vi "TiMicSDK.vi"() -> ()   [LabVIEW 2011]
uses:
  TILLPhotonics/DevID.ctl
panel:
  out "Value":string
  out "error out":errorcluster
  out "command":string
  # "version without z"
  # "*.z=\"1..\"\n*.x=\"...\"\n*.y=\"...\"\n*.f1=\"..\"\n*.turret=\"...\"\njeweils .set werte"
  # "stage.x.set=\"update\" for read"
  # "remember state! arrival time? not to sent new command before arrival!"
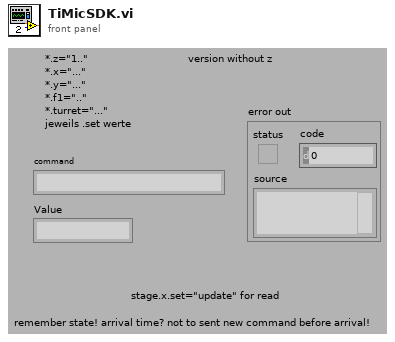
[diagram p1: front panel]
types:
  T1 = enum16{"None/#Datasets", "Clear", "TagValueOf#", "AddValues", "ReadValue", "ChangeValue", "Get all"}
  T2 = typedef "DevID.ctl" = i32
  T3 = enum16{"no error", "missing axis", "missing Z axis", "missing Filter", "iMic not initialized", "no property", "wrong handle", "protocol not finished", "user parameter to long (>32 bits)", "no user parameter handle", "failed to open comport", "failed to initialize"}
  T4 = cluster{bool, "output param":enum16{"no error", "missing axis", "missing Z axis", "missing Filter", "iMic not initialized", "no property", "wrong handle", "protocol not finished", "user parameter to long (>32 bits)", "no user parameter handle", "failed to open comport", "failed to initialize"}, string}
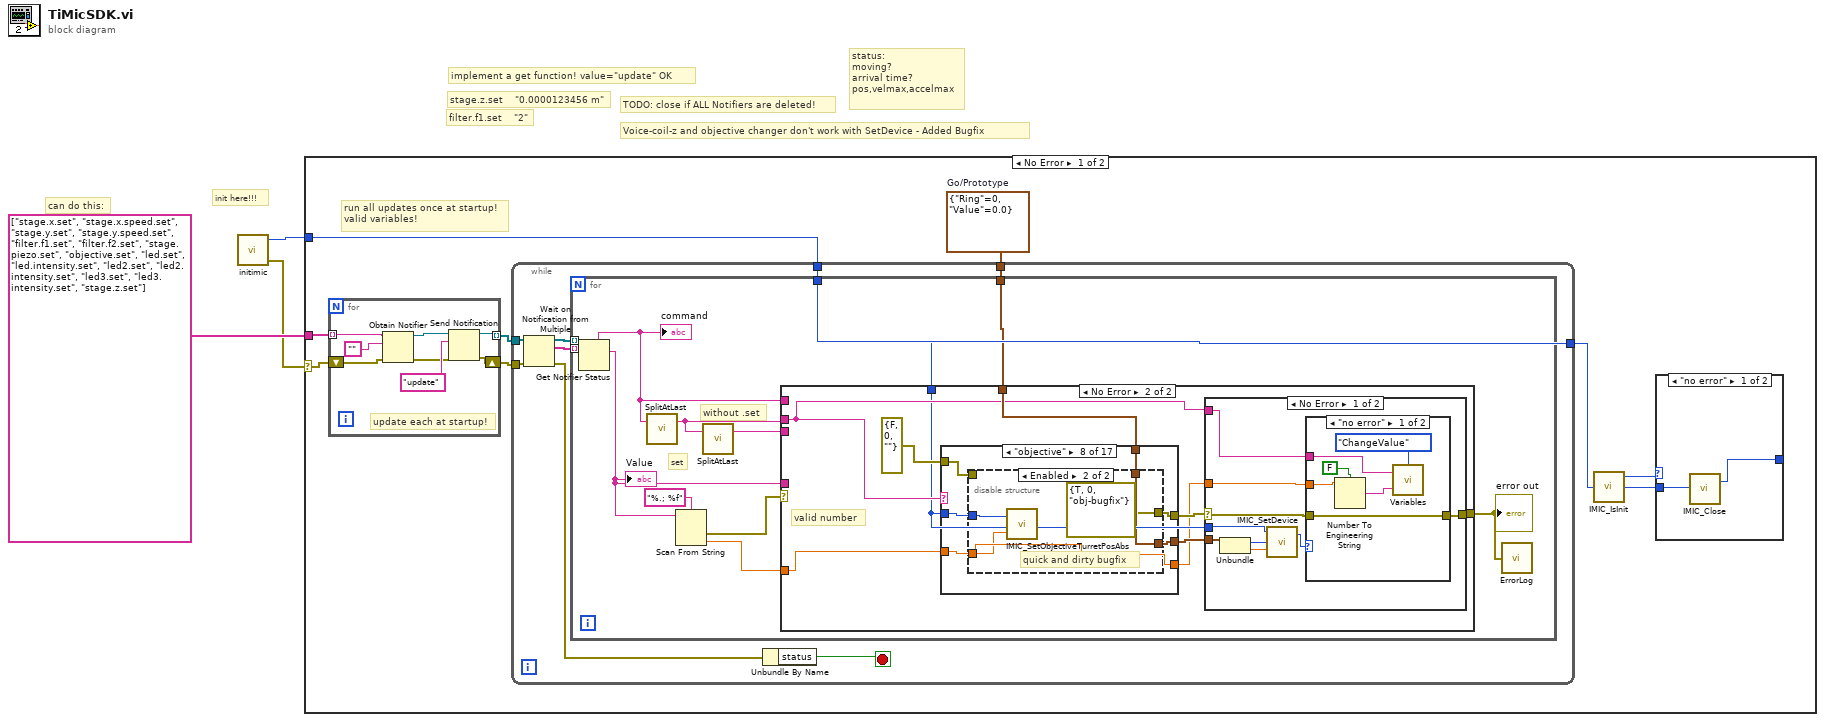
[diagram p0: block diagram]
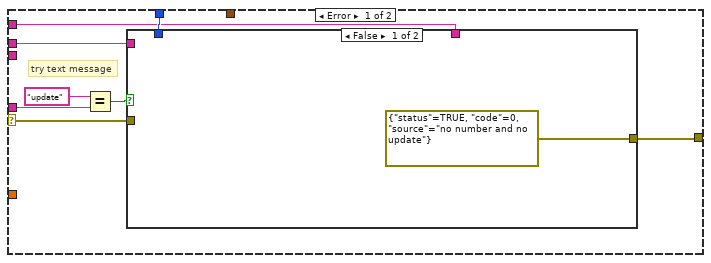
[diagram p3: hidden frame]
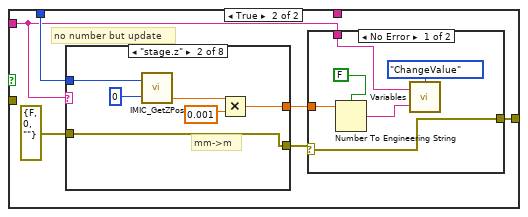
[diagram p4: hidden frame]
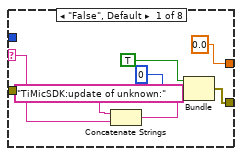
[diagram p6: hidden frame]
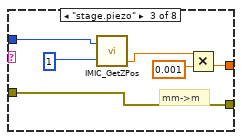
[diagram p7: hidden frame]
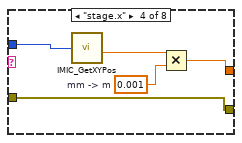
[diagram p8: hidden frame]
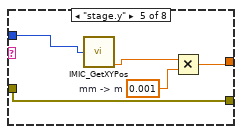
[diagram p9: hidden frame]
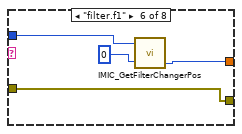
[diagram p10: hidden frame]
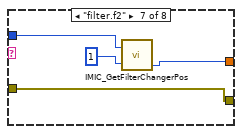
[diagram p11: hidden frame]
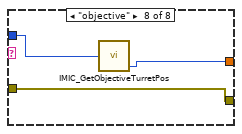
[diagram p12: hidden frame]
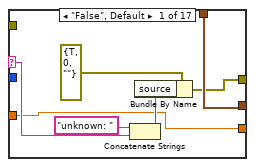
[diagram p13: hidden frame]
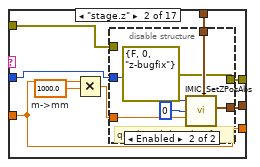
[diagram p14: hidden frame]
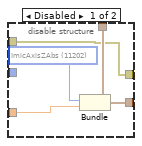
[diagram p15: hidden frame]
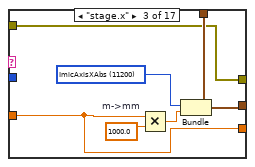
[diagram p16: hidden frame]
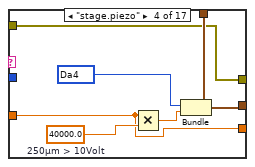
[diagram p17: hidden frame]
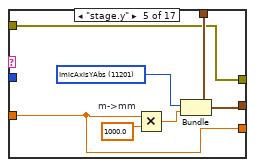
[diagram p18: hidden frame]
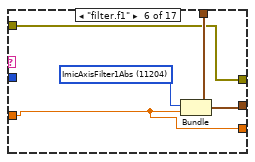
[diagram p19: hidden frame]
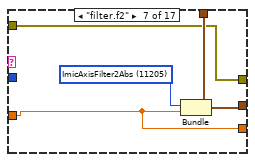
[diagram p20: hidden frame]
diagram:
  # "can do this:"
  # "Voice-coil-z and objective changer don't work with SetDevice - Added Bugfix"
  # "filter.f1.set    \"2\""
  # "status:\nmoving?\narrival time?\npos,velmax,accelmax"
  # "implement a get function! value=\"update\" OK"
  # "TODO: close if ALL Notifiers are deleted!"
  # "init here!!!"
  # "stage.z.set    \"0.0000123456 m\""
  n1 = call "initimic.vi"() -> ("handle"=w3:u64, "error out"=w1:errorcluster)  [unwired: 3 out]
  n2 = case shown="No Error" w1 {
    selector: w1 -> [w4 _]
    tunnel: w3 -> [w12 _]
    tunnel: string[] ["stage.x.set", "stage.x.speed.set", "stage.y.set", "stage.y.speed.set", "filter.f1.set", "filter.f2.set", "stage.piezo.set", "objective.set", "led.set", "led.intensity.set", "led2.set", "led2.intensity.set", "led3.set", "led3.intensity.set", "stage.z.set"] -> [w7 _]
    frame No Error {
      w8 = cluster{"Ring":T2, "Value":dbl} {"Ring"=0, "Value"=0.0}  # Go/Prototype
      # "run all updates once at startup!\nvalid variables!"
      n3 = for {
        tunnel: w7 -> [w20] mode=indexing
        tunnel: [w14] -> w6 mode=indexing
        shift-right: [w13] -> w5
        shift-left: w4 -> [w18]
        # "update each at startup!"
        n4 = Obtain Notifier(name (unnamed)=w20, notification data type="", error in (no error)=w18) -> (notifier out=w16:refnum<notifier>, error out=w15:errorcluster)  [unwired: 1 in, 1 out]
        n5 = Send Notification(notification="update" ("Meldung"), notifier=w16, error in (no error)=w15) -> (notifier out=w14:refnum<notifier>, error out=w13:errorcluster)
      }
      n6 = while {
        tunnel: w6 -> [w26]
        tunnel: w12 -> [w30]
        tunnel: w5 -> [w28]
        tunnel: [w30] -> w10
        tunnel: w8 -> [w29]
        stop <- w31 stop-if-true
        n7 = Wait on Notification from Multiple(0:w26, 3:w28) -> (8:w25:refnum<notifier>[], 9:w24:string[], 11:w27:errorcluster)  [unwired: 3 out]
        n8 = for {
          tunnel: w30 -> [w42]
          tunnel: w29 -> [w41]
          tunnel: w25 -> [w40] mode=indexing
          tunnel: w24 -> [_] mode=indexing
          # "without .set"
          # "set"
          n9 = Get Notifier Status(notifier=w40) -> (notifier name=w39:string, current notification=w33:string)  [unwired: 1 in, 3 out]
          "command" <- w39
          "Value" <- w33
          n10 = call "SplitAtLast.vi"("In-String"=w39) -> ("Front (default)"=w38:string)  [unwired: 1 in, 1 out]
          n11 = Scan From String(format string="%.; %f", input string=w33) -> (error out=w34:errorcluster, output 1=w35:dbl)  [unwired: 2 in, 3 out]
          n12 = call "SplitAtLast.vi"("In-String"=w38) -> ("Front (default)"=w37:string)  [unwired: 1 in, 1 out]
          n13 = case shown="No Error" w34 {
            selector: w34 -> [w48 _]
            tunnel: [w49 w113] -> w32
            tunnel: w42 -> [w50 w107]
            tunnel: w38 -> [w43 w108]
            tunnel: w39 -> [w47 _]
            tunnel: w41 -> [_ w111]
            tunnel: w37 -> [_ _]
            tunnel: w35 -> [_ w106]
            tunnel: w33 -> [w46 _]
            frame Error {
              # "try text message"
              n14 = Equal?(x="update", y=w46) -> (x = y?=w44:bool)
              n15 = case shown="False" w44 {
                tunnel: w50 -> [_ w57]
                tunnel: [errorcluster {"status"=TRUE, "code"=0, "source"="no number and no update"} ("error out") w56] -> w49
                tunnel: w48 -> [_ _]
                tunnel: w47 -> [_ _]
                tunnel: w43 -> [_ w54]
                frame False {
                }
                frame True {
                  # "no number but update"
                  n16 = case shown="\"stage.z\"" w54 {
                    selector: w54 -> [w69 _ _ _ _ _ _ _]
                    tunnel: w57 -> [_ w77 w83 w88 w92 w97 w100 w104]
                    tunnel: [0.0 ("zpos") w73 w79 w85 w90 w95 w99 w103] -> w55
                    tunnel: errorcluster {"status"=FALSE, "code"=0, "source"=""} ("error out") -> [_ w72 w78 w84 w89 w94 w98 w102]
                    tunnel: [w68 w72 w78 w84 w89 w94 w98 w102] -> w52
                    frame "False", Default {
                      n17 = Concatenate Strings("TiMicSDK:update of unknown:" ("source"), w69) -> (w65:string)
                      n18 = Bundle("status"=TRUE, "code"=0, w65) -> (w68:cluster{"status":bool, "code":i32, string})  [unwired: 1 out]
                    }
                    frame "stage.z" {
                      # "mm->m"
                      n19 = call "IMIC_GetZPos.vi"("handle"=w77, "index"=0) -> ("zpos"=w74:dbl)  [unwired: 2 out]
                      n20 = Multiply(x=w74, y=0.001) -> (x*y=w73:dbl)
                    }
                    frame "stage.piezo" {
                      # "mm->m"
                      n21 = call "IMIC_GetZPos.vi"("handle"=w83, "index"=1) -> ("zpos"=w80:dbl)  [unwired: 2 out]
                      n22 = Multiply(x=w80, y=0.001) -> (x*y=w79:dbl)
                    }
                    frame "stage.x" {
                      w86 = 0.001  # mm -> m
                      n23 = call "IMIC_GetXYPos.vi"("handle"=w88) -> ("xpos"=w87:dbl)  [unwired: 3 out]
                      n24 = Multiply(x=w87, y=w86) -> (x*y=w85:dbl)
                    }
                    frame "stage.y" {
                      w93 = 0.001  # mm -> m
                      n25 = call "IMIC_GetXYPos.vi"("handle"=w92) -> ("ypos"=w91:dbl)  [unwired: 3 out]
                      n26 = Multiply(x=w91, y=w93) -> (x*y=w90:dbl)
                    }
                    frame "filter.f1" {
                      n27 = call "IMIC_GetFilterChangerPos.vi"("handle"=w97, "index"=0) -> ("Filter"=w95:i32)  [unwired: 2 out]
                    }
                    frame "filter.f2" {
                      n28 = call "IMIC_GetFilterChangerPos.vi"("handle"=w100, "index"=1) -> ("Filter"=w99:i32)  [unwired: 2 out]
                    }
                    frame "objective" {
                      n29 = call "IMIC_GetObjectiveTurretPos.vi"("handle"=w104) -> ("Objective"=w103:i32)  [unwired: 2 out]
                    }
                  }
                  n30 = case shown="No Error" w52 {
                    selector: w52 -> [w58 w64]
                    tunnel: [w58 w64] -> w56
                    tunnel: w55 -> [w60 _]
                    tunnel: w54 -> [w59 _]
                    frame No Error {
                      n31 = Number To Engineering String(1:FALSE ("use system decimal point (T)"), 4:w60) -> (0:w63:string)  [unwired: 2 out]
                      n32 = call "Variables.vi"("value"=w63, "Tag in"=w59, "Command"=T1."ChangeValue") -> ()  [unwired: 3 out]
                    }
                    frame Error {
                    }
                  }
                }
              }
            }
            frame No Error {
              # "valid number"
              n33 = case shown="\"objective\"" w108 {
                selector: w108 -> [w118 _ _ _ _ _ _ _ _ _ _ _ _ _ _ _ _]
                tunnel: w106 -> [w114 w125 w139 w146 w153 w160 w165 w172 w185 w195 w205 w219 w228 w236 w243 w251 w260]
                tunnel: [w115 w122 w141 w149 w155 w161 w166 w170 w187 w196 w206 w215 w224 w232 w239 w247 w256] -> w109
                tunnel: [w120 w126 w143 w151 w157 w163 w168 w175 w188 w198 w207 w222 w230 w238 w241 w249 w258] -> w110
                tunnel: w111 -> [w120 w127 w144 w152 w158 w164 w169 w173 w186 w197 w208 w221 w229 w237 w240 w248 w257]
                tunnel: errorcluster {"status"=FALSE, "code"=0, "source"=""} ("error in (no error)") -> [_ w123 w141 w149 w155 w161 w166 w171 w187 w196 w206 w215 w224 w232 w239 w247 w256]
                tunnel: w107 -> [_ w121 _ _ _ _ _ w174 _ _ _ _ _ _ _ _ _]
                tunnel: [w114 w125 w139 w146 w153 w160 w165 w172 w185 w195 w205 w216 w225 w233 w242 w250 w259] -> w105
                frame "False", Default {
                  n34 = Concatenate Strings("unknown: ", w118) -> (w117:string)
                  n35 = Bundle By Name(cluster=errorcluster {"status"=TRUE, "code"=0, "source"=""} ("error out"), "source"=w117) -> (w115:errorcluster)
                }
                frame "stage.z" {
                  w128 = 1000.0  # m->mm
                  n36 = Multiply(x=w125, y=w128) -> (x*y=w124:dbl)
                  n37 = disable-structure shown="Enabled" {
                    disable-tunnel: w127 -> [w133 w138]
                    disable-tunnel: [w132 w138] -> w126
                    disable-tunnel: w124 -> [w130 w135]
                    disable-tunnel: w123 -> [w129 _]
                    disable-tunnel: [w129 errorcluster {"status"=FALSE, "code"=0, "source"="z-bugfix"} ("error in (no error)")] -> w122
                    disable-tunnel: w121 -> [_ w136]
                    frame Disabled {
                      w131 = 11202 items=["EndLoop"=-2, "Loop"=-1, "Invalid"=0, "TriggerPolyV"=1, "TriggerCamera"=2, "SyncCamera"=3, "Do1"=1000, "Do2"=1001, "Do3"=1002, "Do4"=1003, "Do5"=1004, "Do6"=1005, "Do7"=1006, "Do8"=1007, "Do9"=1008, "Do10"=1009, "Do11"=1010, "Do12"=1011, "Do13"=1012, "Do14"=1013, "Do15"=1014, "Do16"=1015, "Do17"=1016, "Do18"=1017, "Do19"=1018, "Do20"=1019, "Do21"=1020, "Do22"=1021, "Do23"=1022, "Do24"=1023, "Do_End"=1024, "Da1"=2000, "Da2"=2001, "Da3"=2002, "Da4"=2003, "Da5"=2004, "Da6"=2005, "Da7"=2006, "Da8"=2007, "DaIncr_First"=2008, "Da1Incr"=2100, "Da2Incr"=2101, "Da3Incr"=2102, "Da4Incr"=2103, "Da5Incr"=2104, "Da6Incr"=2105, "Da7Incr"=2106, "Da8Incr"=2107, "Da1Raw"=2200, "Da2Raw"=2201, "Da3Raw"=2202, "Da4Raw"=2203, "Da5Raw"=2204, "Da6Raw"=2205, "Da7Raw"=2206, "Da8Raw"=2207, "Da1RawIncr"=2300, "Da2RawIncr"=2301, "Da3RawIncr"=2302, "Da4RawIncr"=2303, "Da5RawIncr"=2304, "Da6RawIncr"=2305, "Da7RawIncr"=2306, "Da8RawIncr"=2307, "Uart1"=3000, "Uart2"=3001, "Uart3"=3002, "Uart_End"=3003, "Di1"=4000, "Di2"=4001, "Di3"=4002, "Di4"=4003, "Di5"=4004, "Di6"=4005, "Di7"=4006, "Di8"=4007, "Di9"=4008, "Di10"=4009, "Di11"=4010, "Di12"=4011, "Di13"=4012, "Di14"=4013, "Di15"=4014, "Di16"=4015, "Di17"=4016, "Di18"=4017, "Di19"=4018, "Di20"=4019, "Di21"=4020, "Di22"=4021, "Di23"=4022, "Di24"=4023, "Di_End"=4024, "ICU_End"=4025, "LedIllum"=10000, "ImicAxisXRel"=11000, "ImicAxisYRel"=11001, "ImicAxisZRel"=11002, "ImicAxisTurretRel"=11003, "ImicAxisFilter1Rel"=11004, "ImicAxisFilter2Rel"=11005, "ImicAxis_End"=11006, "ImicAxisXAbs"=11200, "ImicAxisYAbs"=11201, "ImicAxisZAbs"=11202, "ImicAxisTurretAbs"=11203, "ImicAxisFilter1Abs"=11204, "ImicAxisFilter2Abs"=11205, "ImicAxisXVel"=11300, "ImicAxisYVel"=11301, "ImicAxisZVel"=11302, "ImicAxisTurretVel"=11303, "ImicAxisFilter1Vel"=11304, "ImicAxisFilter2Vel"=11305, "ImicAxisXMoving"=11400, "ImicAxisYMoving"=11401, "ImicAxisZMoving"=11402, "ImicAxisTurretMoving"=11403, "ImicAxisFilter1Moving"=11404, "ImicAxisFilter2Moving"=11405, "ImicPiezoClip"=12001, "ImicPiezo"=12002, "IMIC_End"=12003] ("DeviceID")
                      n38 = Bundle(cluster=w133, "Ring"=w131, "Value"=w130) -> (w132:cluster{"Ring":T2, "Value":dbl})
                    }
                    frame Enabled {
                      # "quick and dirty bugfix"
                      n39 = call "IMIC_SetZPosAbs.vi"("zpos"=w135, "index"=0, "handle"=w136) -> ()  [unwired: 2 out]
                    }
                  }
                }
                frame "stage.x" {
                  w142 = 11200 items=["EndLoop"=-2, "Loop"=-1, "Invalid"=0, "TriggerPolyV"=1, "TriggerCamera"=2, "SyncCamera"=3, "Do1"=1000, "Do2"=1001, "Do3"=1002, "Do4"=1003, "Do5"=1004, "Do6"=1005, "Do7"=1006, "Do8"=1007, "Do9"=1008, "Do10"=1009, "Do11"=1010, "Do12"=1011, "Do13"=1012, "Do14"=1013, "Do15"=1014, "Do16"=1015, "Do17"=1016, "Do18"=1017, "Do19"=1018, "Do20"=1019, "Do21"=1020, "Do22"=1021, "Do23"=1022, "Do24"=1023, "Do_End"=1024, "Da1"=2000, "Da2"=2001, "Da3"=2002, "Da4"=2003, "Da5"=2004, "Da6"=2005, "Da7"=2006, "Da8"=2007, "DaIncr_First"=2008, "Da1Incr"=2100, "Da2Incr"=2101, "Da3Incr"=2102, "Da4Incr"=2103, "Da5Incr"=2104, "Da6Incr"=2105, "Da7Incr"=2106, "Da8Incr"=2107, "Da1Raw"=2200, "Da2Raw"=2201, "Da3Raw"=2202, "Da4Raw"=2203, "Da5Raw"=2204, "Da6Raw"=2205, "Da7Raw"=2206, "Da8Raw"=2207, "Da1RawIncr"=2300, "Da2RawIncr"=2301, "Da3RawIncr"=2302, "Da4RawIncr"=2303, "Da5RawIncr"=2304, "Da6RawIncr"=2305, "Da7RawIncr"=2306, "Da8RawIncr"=2307, "Uart1"=3000, "Uart2"=3001, "Uart3"=3002, "Uart_End"=3003, "Di1"=4000, "Di2"=4001, "Di3"=4002, "Di4"=4003, "Di5"=4004, "Di6"=4005, "Di7"=4006, "Di8"=4007, "Di9"=4008, "Di10"=4009, "Di11"=4010, "Di12"=4011, "Di13"=4012, "Di14"=4013, "Di15"=4014, "Di16"=4015, "Di17"=4016, "Di18"=4017, "Di19"=4018, "Di20"=4019, "Di21"=4020, "Di22"=4021, "Di23"=4022, "Di24"=4023, "Di_End"=4024, "ICU_End"=4025, "LedIllum"=10000, "ImicAxisXRel"=11000, "ImicAxisYRel"=11001, "ImicAxisZRel"=11002, "ImicAxisTurretRel"=11003, "ImicAxisFilter1Rel"=11004, "ImicAxisFilter2Rel"=11005, "ImicAxis_End"=11006, "ImicAxisXAbs"=11200, "ImicAxisYAbs"=11201, "ImicAxisZAbs"=11202, "ImicAxisTurretAbs"=11203, "ImicAxisFilter1Abs"=11204, "ImicAxisFilter2Abs"=11205, "ImicAxisXVel"=11300, "ImicAxisYVel"=11301, "ImicAxisZVel"=11302, "ImicAxisTurretVel"=11303, "ImicAxisFilter1Vel"=11304, "ImicAxisFilter2Vel"=11305, "ImicAxisXMoving"=11400, "ImicAxisYMoving"=11401, "ImicAxisZMoving"=11402, "ImicAxisTurretMoving"=11403, "ImicAxisFilter1Moving"=11404, "ImicAxisFilter2Moving"=11405, "ImicPiezoClip"=12001, "ImicPiezo"=12002, "IMIC_End"=12003] ("DeviceID")
                  w145 = 1000.0  # m->mm
                  n40 = Multiply(x=w139, y=w145) -> (x*y=w140:dbl)
                  n41 = Bundle(cluster=w144, "Ring"=w142, "Value"=w140) -> (w143:cluster{"Ring":T2, "Value":dbl})
                }
                frame "stage.piezo" {
                  w147 = 40000.0  # 250µm > 10Volt
                  w150 = 2003 items=["EndLoop"=-2, "Loop"=-1, "Invalid"=0, "TriggerPolyV"=1, "TriggerCamera"=2, "SyncCamera"=3, "Do1"=1000, "Do2"=1001, "Do3"=1002, "Do4"=1003, "Do5"=1004, "Do6"=1005, "Do7"=1006, "Do8"=1007, "Do9"=1008, "Do10"=1009, "Do11"=1010, "Do12"=1011, "Do13"=1012, "Do14"=1013, "Do15"=1014, "Do16"=1015, "Do17"=1016, "Do18"=1017, "Do19"=1018, "Do20"=1019, "Do21"=1020, "Do22"=1021, "Do23"=1022, "Do24"=1023, "Do_End"=1024, "Da1"=2000, "Da2"=2001, "Da3"=2002, "Da4"=2003, "Da5"=2004, "Da6"=2005, "Da7"=2006, "Da8"=2007, "DaIncr_First"=2008, "Da1Incr"=2100, "Da2Incr"=2101, "Da3Incr"=2102, "Da4Incr"=2103, "Da5Incr"=2104, "Da6Incr"=2105, "Da7Incr"=2106, "Da8Incr"=2107, "Da1Raw"=2200, "Da2Raw"=2201, "Da3Raw"=2202, "Da4Raw"=2203, "Da5Raw"=2204, "Da6Raw"=2205, "Da7Raw"=2206, "Da8Raw"=2207, "Da1RawIncr"=2300, "Da2RawIncr"=2301, "Da3RawIncr"=2302, "Da4RawIncr"=2303, "Da5RawIncr"=2304, "Da6RawIncr"=2305, "Da7RawIncr"=2306, "Da8RawIncr"=2307, "Uart1"=3000, "Uart2"=3001, "Uart3"=3002, "Uart_End"=3003, "Di1"=4000, "Di2"=4001, "Di3"=4002, "Di4"=4003, "Di5"=4004, "Di6"=4005, "Di7"=4006, "Di8"=4007, "Di9"=4008, "Di10"=4009, "Di11"=4010, "Di12"=4011, "Di13"=4012, "Di14"=4013, "Di15"=4014, "Di16"=4015, "Di17"=4016, "Di18"=4017, "Di19"=4018, "Di20"=4019, "Di21"=4020, "Di22"=4021, "Di23"=4022, "Di24"=4023, "Di_End"=4024, "ICU_End"=4025, "LedIllum"=10000, "ImicAxisXRel"=11000, "ImicAxisYRel"=11001, "ImicAxisZRel"=11002, "ImicAxisTurretRel"=11003, "ImicAxisFilter1Rel"=11004, "ImicAxisFilter2Rel"=11005, "ImicAxis_End"=11006, "ImicAxisXAbs"=11200, "ImicAxisYAbs"=11201, "ImicAxisZAbs"=11202, "ImicAxisTurretAbs"=11203, "ImicAxisFilter1Abs"=11204, "ImicAxisFilter2Abs"=11205, "ImicAxisXVel"=11300, "ImicAxisYVel"=11301, "ImicAxisZVel"=11302, "ImicAxisTurretVel"=11303, "ImicAxisFilter1Vel"=11304, "ImicAxisFilter2Vel"=11305, "ImicAxisXMoving"=11400, "ImicAxisYMoving"=11401, "ImicAxisZMoving"=11402, "ImicAxisTurretMoving"=11403, "ImicAxisFilter1Moving"=11404, "ImicAxisFilter2Moving"=11405, "ImicPiezoClip"=12001, "ImicPiezo"=12002, "IMIC_End"=12003] ("DeviceID")
                  n42 = Multiply(x=w146, y=w147) -> (x*y=w148:dbl)
                  n43 = Bundle(cluster=w152, "Ring"=w150, "Value"=w148) -> (w151:cluster{"Ring":T2, "Value":dbl})
                }
                frame "stage.y" {
                  w156 = 11201 items=["EndLoop"=-2, "Loop"=-1, "Invalid"=0, "TriggerPolyV"=1, "TriggerCamera"=2, "SyncCamera"=3, "Do1"=1000, "Do2"=1001, "Do3"=1002, "Do4"=1003, "Do5"=1004, "Do6"=1005, "Do7"=1006, "Do8"=1007, "Do9"=1008, "Do10"=1009, "Do11"=1010, "Do12"=1011, "Do13"=1012, "Do14"=1013, "Do15"=1014, "Do16"=1015, "Do17"=1016, "Do18"=1017, "Do19"=1018, "Do20"=1019, "Do21"=1020, "Do22"=1021, "Do23"=1022, "Do24"=1023, "Do_End"=1024, "Da1"=2000, "Da2"=2001, "Da3"=2002, "Da4"=2003, "Da5"=2004, "Da6"=2005, "Da7"=2006, "Da8"=2007, "DaIncr_First"=2008, "Da1Incr"=2100, "Da2Incr"=2101, "Da3Incr"=2102, "Da4Incr"=2103, "Da5Incr"=2104, "Da6Incr"=2105, "Da7Incr"=2106, "Da8Incr"=2107, "Da1Raw"=2200, "Da2Raw"=2201, "Da3Raw"=2202, "Da4Raw"=2203, "Da5Raw"=2204, "Da6Raw"=2205, "Da7Raw"=2206, "Da8Raw"=2207, "Da1RawIncr"=2300, "Da2RawIncr"=2301, "Da3RawIncr"=2302, "Da4RawIncr"=2303, "Da5RawIncr"=2304, "Da6RawIncr"=2305, "Da7RawIncr"=2306, "Da8RawIncr"=2307, "Uart1"=3000, "Uart2"=3001, "Uart3"=3002, "Uart_End"=3003, "Di1"=4000, "Di2"=4001, "Di3"=4002, "Di4"=4003, "Di5"=4004, "Di6"=4005, "Di7"=4006, "Di8"=4007, "Di9"=4008, "Di10"=4009, "Di11"=4010, "Di12"=4011, "Di13"=4012, "Di14"=4013, "Di15"=4014, "Di16"=4015, "Di17"=4016, "Di18"=4017, "Di19"=4018, "Di20"=4019, "Di21"=4020, "Di22"=4021, "Di23"=4022, "Di24"=4023, "Di_End"=4024, "ICU_End"=4025, "LedIllum"=10000, "ImicAxisXRel"=11000, "ImicAxisYRel"=11001, "ImicAxisZRel"=11002, "ImicAxisTurretRel"=11003, "ImicAxisFilter1Rel"=11004, "ImicAxisFilter2Rel"=11005, "ImicAxis_End"=11006, "ImicAxisXAbs"=11200, "ImicAxisYAbs"=11201, "ImicAxisZAbs"=11202, "ImicAxisTurretAbs"=11203, "ImicAxisFilter1Abs"=11204, "ImicAxisFilter2Abs"=11205, "ImicAxisXVel"=11300, "ImicAxisYVel"=11301, "ImicAxisZVel"=11302, "ImicAxisTurretVel"=11303, "ImicAxisFilter1Vel"=11304, "ImicAxisFilter2Vel"=11305, "ImicAxisXMoving"=11400, "ImicAxisYMoving"=11401, "ImicAxisZMoving"=11402, "ImicAxisTurretMoving"=11403, "ImicAxisFilter1Moving"=11404, "ImicAxisFilter2Moving"=11405, "ImicPiezoClip"=12001, "ImicPiezo"=12002, "IMIC_End"=12003] ("DeviceID")
                  w159 = 1000.0  # m->mm
                  n44 = Multiply(x=w153, y=w159) -> (x*y=w154:dbl)
                  n45 = Bundle(cluster=w158, "Ring"=w156, "Value"=w154) -> (w157:cluster{"Ring":T2, "Value":dbl})
                }
                frame "filter.f1" {
                  w162 = 11204 items=["EndLoop"=-2, "Loop"=-1, "Invalid"=0, "TriggerPolyV"=1, "TriggerCamera"=2, "SyncCamera"=3, "Do1"=1000, "Do2"=1001, "Do3"=1002, "Do4"=1003, "Do5"=1004, "Do6"=1005, "Do7"=1006, "Do8"=1007, "Do9"=1008, "Do10"=1009, "Do11"=1010, "Do12"=1011, "Do13"=1012, "Do14"=1013, "Do15"=1014, "Do16"=1015, "Do17"=1016, "Do18"=1017, "Do19"=1018, "Do20"=1019, "Do21"=1020, "Do22"=1021, "Do23"=1022, "Do24"=1023, "Do_End"=1024, "Da1"=2000, "Da2"=2001, "Da3"=2002, "Da4"=2003, "Da5"=2004, "Da6"=2005, "Da7"=2006, "Da8"=2007, "DaIncr_First"=2008, "Da1Incr"=2100, "Da2Incr"=2101, "Da3Incr"=2102, "Da4Incr"=2103, "Da5Incr"=2104, "Da6Incr"=2105, "Da7Incr"=2106, "Da8Incr"=2107, "Da1Raw"=2200, "Da2Raw"=2201, "Da3Raw"=2202, "Da4Raw"=2203, "Da5Raw"=2204, "Da6Raw"=2205, "Da7Raw"=2206, "Da8Raw"=2207, "Da1RawIncr"=2300, "Da2RawIncr"=2301, "Da3RawIncr"=2302, "Da4RawIncr"=2303, "Da5RawIncr"=2304, "Da6RawIncr"=2305, "Da7RawIncr"=2306, "Da8RawIncr"=2307, "Uart1"=3000, "Uart2"=3001, "Uart3"=3002, "Uart_End"=3003, "Di1"=4000, "Di2"=4001, "Di3"=4002, "Di4"=4003, "Di5"=4004, "Di6"=4005, "Di7"=4006, "Di8"=4007, "Di9"=4008, "Di10"=4009, "Di11"=4010, "Di12"=4011, "Di13"=4012, "Di14"=4013, "Di15"=4014, "Di16"=4015, "Di17"=4016, "Di18"=4017, "Di19"=4018, "Di20"=4019, "Di21"=4020, "Di22"=4021, "Di23"=4022, "Di24"=4023, "Di_End"=4024, "ICU_End"=4025, "LedIllum"=10000, "ImicAxisXRel"=11000, "ImicAxisYRel"=11001, "ImicAxisZRel"=11002, "ImicAxisTurretRel"=11003, "ImicAxisFilter1Rel"=11004, "ImicAxisFilter2Rel"=11005, "ImicAxis_End"=11006, "ImicAxisXAbs"=11200, "ImicAxisYAbs"=11201, "ImicAxisZAbs"=11202, "ImicAxisTurretAbs"=11203, "ImicAxisFilter1Abs"=11204, "ImicAxisFilter2Abs"=11205, "ImicAxisXVel"=11300, "ImicAxisYVel"=11301, "ImicAxisZVel"=11302, "ImicAxisTurretVel"=11303, "ImicAxisFilter1Vel"=11304, "ImicAxisFilter2Vel"=11305, "ImicAxisXMoving"=11400, "ImicAxisYMoving"=11401, "ImicAxisZMoving"=11402, "ImicAxisTurretMoving"=11403, "ImicAxisFilter1Moving"=11404, "ImicAxisFilter2Moving"=11405, "ImicPiezoClip"=12001, "ImicPiezo"=12002, "IMIC_End"=12003] ("DeviceID")
                  n46 = Bundle(cluster=w164, "Ring"=w162, "Value"=w160) -> (w163:cluster{"Ring":T2, "Value":dbl})
                }
                frame "filter.f2" {
                  w167 = 11205 items=["EndLoop"=-2, "Loop"=-1, "Invalid"=0, "TriggerPolyV"=1, "TriggerCamera"=2, "SyncCamera"=3, "Do1"=1000, "Do2"=1001, "Do3"=1002, "Do4"=1003, "Do5"=1004, "Do6"=1005, "Do7"=1006, "Do8"=1007, "Do9"=1008, "Do10"=1009, "Do11"=1010, "Do12"=1011, "Do13"=1012, "Do14"=1013, "Do15"=1014, "Do16"=1015, "Do17"=1016, "Do18"=1017, "Do19"=1018, "Do20"=1019, "Do21"=1020, "Do22"=1021, "Do23"=1022, "Do24"=1023, "Do_End"=1024, "Da1"=2000, "Da2"=2001, "Da3"=2002, "Da4"=2003, "Da5"=2004, "Da6"=2005, "Da7"=2006, "Da8"=2007, "DaIncr_First"=2008, "Da1Incr"=2100, "Da2Incr"=2101, "Da3Incr"=2102, "Da4Incr"=2103, "Da5Incr"=2104, "Da6Incr"=2105, "Da7Incr"=2106, "Da8Incr"=2107, "Da1Raw"=2200, "Da2Raw"=2201, "Da3Raw"=2202, "Da4Raw"=2203, "Da5Raw"=2204, "Da6Raw"=2205, "Da7Raw"=2206, "Da8Raw"=2207, "Da1RawIncr"=2300, "Da2RawIncr"=2301, "Da3RawIncr"=2302, "Da4RawIncr"=2303, "Da5RawIncr"=2304, "Da6RawIncr"=2305, "Da7RawIncr"=2306, "Da8RawIncr"=2307, "Uart1"=3000, "Uart2"=3001, "Uart3"=3002, "Uart_End"=3003, "Di1"=4000, "Di2"=4001, "Di3"=4002, "Di4"=4003, "Di5"=4004, "Di6"=4005, "Di7"=4006, "Di8"=4007, "Di9"=4008, "Di10"=4009, "Di11"=4010, "Di12"=4011, "Di13"=4012, "Di14"=4013, "Di15"=4014, "Di16"=4015, "Di17"=4016, "Di18"=4017, "Di19"=4018, "Di20"=4019, "Di21"=4020, "Di22"=4021, "Di23"=4022, "Di24"=4023, "Di_End"=4024, "ICU_End"=4025, "LedIllum"=10000, "ImicAxisXRel"=11000, "ImicAxisYRel"=11001, "ImicAxisZRel"=11002, "ImicAxisTurretRel"=11003, "ImicAxisFilter1Rel"=11004, "ImicAxisFilter2Rel"=11005, "ImicAxis_End"=11006, "ImicAxisXAbs"=11200, "ImicAxisYAbs"=11201, "ImicAxisZAbs"=11202, "ImicAxisTurretAbs"=11203, "ImicAxisFilter1Abs"=11204, "ImicAxisFilter2Abs"=11205, "ImicAxisXVel"=11300, "ImicAxisYVel"=11301, "ImicAxisZVel"=11302, "ImicAxisTurretVel"=11303, "ImicAxisFilter1Vel"=11304, "ImicAxisFilter2Vel"=11305, "ImicAxisXMoving"=11400, "ImicAxisYMoving"=11401, "ImicAxisZMoving"=11402, "ImicAxisTurretMoving"=11403, "ImicAxisFilter1Moving"=11404, "ImicAxisFilter2Moving"=11405, "ImicPiezoClip"=12001, "ImicPiezo"=12002, "IMIC_End"=12003] ("DeviceID")
                  n47 = Bundle(cluster=w169, "Ring"=w167, "Value"=w165) -> (w168:cluster{"Ring":T2, "Value":dbl})
                }
                frame "objective" {
                  n48 = disable-structure shown="Enabled" {
                    disable-tunnel: [w179 w182] -> w175
                    disable-tunnel: w174 -> [_ w184]
                    disable-tunnel: w173 -> [w178 w182]
                    disable-tunnel: w172 -> [w177 w183]
                    disable-tunnel: w171 -> [w176 _]
                    disable-tunnel: [w176 errorcluster {"status"=TRUE, "code"=0, "source"="obj-bugfix"} ("error in (no error)")] -> w170
                    frame Disabled {
                      w180 = 11203 items=["EndLoop"=-2, "Loop"=-1, "Invalid"=0, "TriggerPolyV"=1, "TriggerCamera"=2, "SyncCamera"=3, "Do1"=1000, "Do2"=1001, "Do3"=1002, "Do4"=1003, "Do5"=1004, "Do6"=1005, "Do7"=1006, "Do8"=1007, "Do9"=1008, "Do10"=1009, "Do11"=1010, "Do12"=1011, "Do13"=1012, "Do14"=1013, "Do15"=1014, "Do16"=1015, "Do17"=1016, "Do18"=1017, "Do19"=1018, "Do20"=1019, "Do21"=1020, "Do22"=1021, "Do23"=1022, "Do24"=1023, "Do_End"=1024, "Da1"=2000, "Da2"=2001, "Da3"=2002, "Da4"=2003, "Da5"=2004, "Da6"=2005, "Da7"=2006, "Da8"=2007, "DaIncr_First"=2008, "Da1Incr"=2100, "Da2Incr"=2101, "Da3Incr"=2102, "Da4Incr"=2103, "Da5Incr"=2104, "Da6Incr"=2105, "Da7Incr"=2106, "Da8Incr"=2107, "Da1Raw"=2200, "Da2Raw"=2201, "Da3Raw"=2202, "Da4Raw"=2203, "Da5Raw"=2204, "Da6Raw"=2205, "Da7Raw"=2206, "Da8Raw"=2207, "Da1RawIncr"=2300, "Da2RawIncr"=2301, "Da3RawIncr"=2302, "Da4RawIncr"=2303, "Da5RawIncr"=2304, "Da6RawIncr"=2305, "Da7RawIncr"=2306, "Da8RawIncr"=2307, "Uart1"=3000, "Uart2"=3001, "Uart3"=3002, "Uart_End"=3003, "Di1"=4000, "Di2"=4001, "Di3"=4002, "Di4"=4003, "Di5"=4004, "Di6"=4005, "Di7"=4006, "Di8"=4007, "Di9"=4008, "Di10"=4009, "Di11"=4010, "Di12"=4011, "Di13"=4012, "Di14"=4013, "Di15"=4014, "Di16"=4015, "Di17"=4016, "Di18"=4017, "Di19"=4018, "Di20"=4019, "Di21"=4020, "Di22"=4021, "Di23"=4022, "Di24"=4023, "Di_End"=4024, "ICU_End"=4025, "LedIllum"=10000, "ImicAxisXRel"=11000, "ImicAxisYRel"=11001, "ImicAxisZRel"=11002, "ImicAxisTurretRel"=11003, "ImicAxisFilter1Rel"=11004, "ImicAxisFilter2Rel"=11005, "ImicAxis_End"=11006, "ImicAxisXAbs"=11200, "ImicAxisYAbs"=11201, "ImicAxisZAbs"=11202, "ImicAxisTurretAbs"=11203, "ImicAxisFilter1Abs"=11204, "ImicAxisFilter2Abs"=11205, "ImicAxisXVel"=11300, "ImicAxisYVel"=11301, "ImicAxisZVel"=11302, "ImicAxisTurretVel"=11303, "ImicAxisFilter1Vel"=11304, "ImicAxisFilter2Vel"=11305, "ImicAxisXMoving"=11400, "ImicAxisYMoving"=11401, "ImicAxisZMoving"=11402, "ImicAxisTurretMoving"=11403, "ImicAxisFilter1Moving"=11404, "ImicAxisFilter2Moving"=11405, "ImicPiezoClip"=12001, "ImicPiezo"=12002, "IMIC_End"=12003] ("DeviceID")
                      n49 = Bundle(cluster=w178, "Ring"=w180, "Value"=w177) -> (w179:cluster{"Ring":T2, "Value":dbl})
                    }
                    frame Enabled {
                      # "quick and dirty bugfix"
                      n50 = call "IMIC_SetObjectiveTurretPosAbs.vi"("ObjectivePosAbs"=w183, "handle"=w184) -> ()  [unwired: 2 out]
                    }
                  }
                }
                frame "stage.z.speed" {
                  w194 = 1000.0  # m->mm
                  w193 = 11302 items=["EndLoop"=-2, "Loop"=-1, "Invalid"=0, "TriggerPolyV"=1, "TriggerCamera"=2, "SyncCamera"=3, "Do1"=1000, "Do2"=1001, "Do3"=1002, "Do4"=1003, "Do5"=1004, "Do6"=1005, "Do7"=1006, "Do8"=1007, "Do9"=1008, "Do10"=1009, "Do11"=1010, "Do12"=1011, "Do13"=1012, "Do14"=1013, "Do15"=1014, "Do16"=1015, "Do17"=1016, "Do18"=1017, "Do19"=1018, "Do20"=1019, "Do21"=1020, "Do22"=1021, "Do23"=1022, "Do24"=1023, "Do_End"=1024, "Da1"=2000, "Da2"=2001, "Da3"=2002, "Da4"=2003, "Da5"=2004, "Da6"=2005, "Da7"=2006, "Da8"=2007, "DaIncr_First"=2008, "Da1Incr"=2100, "Da2Incr"=2101, "Da3Incr"=2102, "Da4Incr"=2103, "Da5Incr"=2104, "Da6Incr"=2105, "Da7Incr"=2106, "Da8Incr"=2107, "Da1Raw"=2200, "Da2Raw"=2201, "Da3Raw"=2202, "Da4Raw"=2203, "Da5Raw"=2204, "Da6Raw"=2205, "Da7Raw"=2206, "Da8Raw"=2207, "Da1RawIncr"=2300, "Da2RawIncr"=2301, "Da3RawIncr"=2302, "Da4RawIncr"=2303, "Da5RawIncr"=2304, "Da6RawIncr"=2305, "Da7RawIncr"=2306, "Da8RawIncr"=2307, "Uart1"=3000, "Uart2"=3001, "Uart3"=3002, "Uart_End"=3003, "Di1"=4000, "Di2"=4001, "Di3"=4002, "Di4"=4003, "Di5"=4004, "Di6"=4005, "Di7"=4006, "Di8"=4007, "Di9"=4008, "Di10"=4009, "Di11"=4010, "Di12"=4011, "Di13"=4012, "Di14"=4013, "Di15"=4014, "Di16"=4015, "Di17"=4016, "Di18"=4017, "Di19"=4018, "Di20"=4019, "Di21"=4020, "Di22"=4021, "Di23"=4022, "Di24"=4023, "Di_End"=4024, "ICU_End"=4025, "LedIllum"=10000, "ImicAxisXRel"=11000, "ImicAxisYRel"=11001, "ImicAxisZRel"=11002, "ImicAxisTurretRel"=11003, "ImicAxisFilter1Rel"=11004, "ImicAxisFilter2Rel"=11005, "ImicAxis_End"=11006, "ImicAxisXAbs"=11200, "ImicAxisYAbs"=11201, "ImicAxisZAbs"=11202, "ImicAxisTurretAbs"=11203, "ImicAxisFilter1Abs"=11204, "ImicAxisFilter2Abs"=11205, "ImicAxisXVel"=11300, "ImicAxisYVel"=11301, "ImicAxisZVel"=11302, "ImicAxisTurretVel"=11303, "ImicAxisFilter1Vel"=11304, "ImicAxisFilter2Vel"=11305, "ImicAxisXMoving"=11400, "ImicAxisYMoving"=11401, "ImicAxisZMoving"=11402, "ImicAxisTurretMoving"=11403, "ImicAxisFilter1Moving"=11404, "ImicAxisFilter2Moving"=11405, "ImicPiezoClip"=12001, "ImicPiezo"=12002, "IMIC_End"=12003] ("DeviceID")
                  n51 = Not Equal To 0?(x=w185) -> (x != 0?=w190:bool)
                  n52 = Select(t=w185, s=w190, f=0.001) -> (s? t:f=w189:dbl)
                  n53 = Multiply(x=w189, y=w194) -> (x*y=w192:dbl)
                  n54 = Bundle(cluster=w186, "Ring"=w193, "Value"=w192) -> (w188:cluster{"Ring":T2, "Value":dbl})
                }
                frame "stage.x.speed" {
                  w204 = 1000.0  # m->mm
                  w203 = 11300 items=["EndLoop"=-2, "Loop"=-1, "Invalid"=0, "TriggerPolyV"=1, "TriggerCamera"=2, "SyncCamera"=3, "Do1"=1000, "Do2"=1001, "Do3"=1002, "Do4"=1003, "Do5"=1004, "Do6"=1005, "Do7"=1006, "Do8"=1007, "Do9"=1008, "Do10"=1009, "Do11"=1010, "Do12"=1011, "Do13"=1012, "Do14"=1013, "Do15"=1014, "Do16"=1015, "Do17"=1016, "Do18"=1017, "Do19"=1018, "Do20"=1019, "Do21"=1020, "Do22"=1021, "Do23"=1022, "Do24"=1023, "Do_End"=1024, "Da1"=2000, "Da2"=2001, "Da3"=2002, "Da4"=2003, "Da5"=2004, "Da6"=2005, "Da7"=2006, "Da8"=2007, "DaIncr_First"=2008, "Da1Incr"=2100, "Da2Incr"=2101, "Da3Incr"=2102, "Da4Incr"=2103, "Da5Incr"=2104, "Da6Incr"=2105, "Da7Incr"=2106, "Da8Incr"=2107, "Da1Raw"=2200, "Da2Raw"=2201, "Da3Raw"=2202, "Da4Raw"=2203, "Da5Raw"=2204, "Da6Raw"=2205, "Da7Raw"=2206, "Da8Raw"=2207, "Da1RawIncr"=2300, "Da2RawIncr"=2301, "Da3RawIncr"=2302, "Da4RawIncr"=2303, "Da5RawIncr"=2304, "Da6RawIncr"=2305, "Da7RawIncr"=2306, "Da8RawIncr"=2307, "Uart1"=3000, "Uart2"=3001, "Uart3"=3002, "Uart_End"=3003, "Di1"=4000, "Di2"=4001, "Di3"=4002, "Di4"=4003, "Di5"=4004, "Di6"=4005, "Di7"=4006, "Di8"=4007, "Di9"=4008, "Di10"=4009, "Di11"=4010, "Di12"=4011, "Di13"=4012, "Di14"=4013, "Di15"=4014, "Di16"=4015, "Di17"=4016, "Di18"=4017, "Di19"=4018, "Di20"=4019, "Di21"=4020, "Di22"=4021, "Di23"=4022, "Di24"=4023, "Di_End"=4024, "ICU_End"=4025, "LedIllum"=10000, "ImicAxisXRel"=11000, "ImicAxisYRel"=11001, "ImicAxisZRel"=11002, "ImicAxisTurretRel"=11003, "ImicAxisFilter1Rel"=11004, "ImicAxisFilter2Rel"=11005, "ImicAxis_End"=11006, "ImicAxisXAbs"=11200, "ImicAxisYAbs"=11201, "ImicAxisZAbs"=11202, "ImicAxisTurretAbs"=11203, "ImicAxisFilter1Abs"=11204, "ImicAxisFilter2Abs"=11205, "ImicAxisXVel"=11300, "ImicAxisYVel"=11301, "ImicAxisZVel"=11302, "ImicAxisTurretVel"=11303, "ImicAxisFilter1Vel"=11304, "ImicAxisFilter2Vel"=11305, "ImicAxisXMoving"=11400, "ImicAxisYMoving"=11401, "ImicAxisZMoving"=11402, "ImicAxisTurretMoving"=11403, "ImicAxisFilter1Moving"=11404, "ImicAxisFilter2Moving"=11405, "ImicPiezoClip"=12001, "ImicPiezo"=12002, "IMIC_End"=12003] ("DeviceID")
                  n55 = Not Equal To 0?(x=w195) -> (x != 0?=w200:bool)
                  n56 = Select(t=w195, s=w200, f=0.02) -> (s? t:f=w199:dbl)
                  n57 = Multiply(x=w199, y=w204) -> (x*y=w202:dbl)
                  n58 = Bundle(cluster=w197, "Ring"=w203, "Value"=w202) -> (w198:cluster{"Ring":T2, "Value":dbl})
                }
                frame "stage.y.speed" {
                  w214 = 1000.0  # m->mm
                  w213 = 11301 items=["EndLoop"=-2, "Loop"=-1, "Invalid"=0, "TriggerPolyV"=1, "TriggerCamera"=2, "SyncCamera"=3, "Do1"=1000, "Do2"=1001, "Do3"=1002, "Do4"=1003, "Do5"=1004, "Do6"=1005, "Do7"=1006, "Do8"=1007, "Do9"=1008, "Do10"=1009, "Do11"=1010, "Do12"=1011, "Do13"=1012, "Do14"=1013, "Do15"=1014, "Do16"=1015, "Do17"=1016, "Do18"=1017, "Do19"=1018, "Do20"=1019, "Do21"=1020, "Do22"=1021, "Do23"=1022, "Do24"=1023, "Do_End"=1024, "Da1"=2000, "Da2"=2001, "Da3"=2002, "Da4"=2003, "Da5"=2004, "Da6"=2005, "Da7"=2006, "Da8"=2007, "DaIncr_First"=2008, "Da1Incr"=2100, "Da2Incr"=2101, "Da3Incr"=2102, "Da4Incr"=2103, "Da5Incr"=2104, "Da6Incr"=2105, "Da7Incr"=2106, "Da8Incr"=2107, "Da1Raw"=2200, "Da2Raw"=2201, "Da3Raw"=2202, "Da4Raw"=2203, "Da5Raw"=2204, "Da6Raw"=2205, "Da7Raw"=2206, "Da8Raw"=2207, "Da1RawIncr"=2300, "Da2RawIncr"=2301, "Da3RawIncr"=2302, "Da4RawIncr"=2303, "Da5RawIncr"=2304, "Da6RawIncr"=2305, "Da7RawIncr"=2306, "Da8RawIncr"=2307, "Uart1"=3000, "Uart2"=3001, "Uart3"=3002, "Uart_End"=3003, "Di1"=4000, "Di2"=4001, "Di3"=4002, "Di4"=4003, "Di5"=4004, "Di6"=4005, "Di7"=4006, "Di8"=4007, "Di9"=4008, "Di10"=4009, "Di11"=4010, "Di12"=4011, "Di13"=4012, "Di14"=4013, "Di15"=4014, "Di16"=4015, "Di17"=4016, "Di18"=4017, "Di19"=4018, "Di20"=4019, "Di21"=4020, "Di22"=4021, "Di23"=4022, "Di24"=4023, "Di_End"=4024, "ICU_End"=4025, "LedIllum"=10000, "ImicAxisXRel"=11000, "ImicAxisYRel"=11001, "ImicAxisZRel"=11002, "ImicAxisTurretRel"=11003, "ImicAxisFilter1Rel"=11004, "ImicAxisFilter2Rel"=11005, "ImicAxis_End"=11006, "ImicAxisXAbs"=11200, "ImicAxisYAbs"=11201, "ImicAxisZAbs"=11202, "ImicAxisTurretAbs"=11203, "ImicAxisFilter1Abs"=11204, "ImicAxisFilter2Abs"=11205, "ImicAxisXVel"=11300, "ImicAxisYVel"=11301, "ImicAxisZVel"=11302, "ImicAxisTurretVel"=11303, "ImicAxisFilter1Vel"=11304, "ImicAxisFilter2Vel"=11305, "ImicAxisXMoving"=11400, "ImicAxisYMoving"=11401, "ImicAxisZMoving"=11402, "ImicAxisTurretMoving"=11403, "ImicAxisFilter1Moving"=11404, "ImicAxisFilter2Moving"=11405, "ImicPiezoClip"=12001, "ImicPiezo"=12002, "IMIC_End"=12003] ("DeviceID")
                  n59 = Not Equal To 0?(x=w205) -> (x != 0?=w210:bool)
                  n60 = Select(t=w205, s=w210, f=0.02) -> (s? t:f=w211:dbl)
                  n61 = Multiply(x=w211, y=w214) -> (x*y=w212:dbl)
                  n62 = Bundle(cluster=w208, "Ring"=w213, "Value"=w212) -> (w207:cluster{"Ring":T2, "Value":dbl})
                }
                frame "led" {
                  w220 = 1025 items=["EndLoop"=-2, "Loop"=-1, "Invalid"=0, "TriggerPolyV"=1, "TriggerCamera"=2, "SyncCamera"=3, "Do1"=1000, "Do2"=1001, "Do3"=1002, "Do4"=1003, "Do5"=1004, "Do6"=1005, "Do7"=1006, "Do8"=1007, "Do9"=1008, "Do10"=1009, "Do11"=1010, "Do12"=1011, "Do13"=1012, "Do14"=1013, "Do15"=1014, "Do16"=1015, "Do17"=1016, "Do18"=1017, "Do19"=1018, "Do20"=1019, "Do21"=1020, "Do22"=1021, "Do23"=1022, "Do24"=1023, "Do25"=1024, "Do26"=1025, "Da1"=2000, "Da2"=2001, "Da3"=2002, "Da4"=2003, "Da5"=2004, "Da6"=2005, "Da7"=2006, "Da8"=2007, "DaIncr_First"=2008, "Da1Incr"=2100, "Da2Incr"=2101, "Da3Incr"=2102, "Da4Incr"=2103, "Da5Incr"=2104, "Da6Incr"=2105, "Da7Incr"=2106, "Da8Incr"=2107, "Da1Raw"=2200, "Da2Raw"=2201, "Da3Raw"=2202, "Da4Raw"=2203, "Da5Raw"=2204, "Da6Raw"=2205, "Da7Raw"=2206, "Da8Raw"=2207, "Da1RawIncr"=2300, "Da2RawIncr"=2301, "Da3RawIncr"=2302, "Da4RawIncr"=2303, "Da5RawIncr"=2304, "Da6RawIncr"=2305, "Da7RawIncr"=2306, "Da8RawIncr"=2307, "Uart1"=3000, "Uart2"=3001, "Uart3"=3002, "Uart_End"=3003, "Di1"=4000, "Di2"=4001, "Di3"=4002, "Di4"=4003, "Di5"=4004, "Di6"=4005, "Di7"=4006, "Di8"=4007, "Di9"=4008, "Di10"=4009, "Di11"=4010, "Di12"=4011, "Di13"=4012, "Di14"=4013, "Di15"=4014, "Di16"=4015, "Di17"=4016, "Di18"=4017, "Di19"=4018, "Di20"=4019, "Di21"=4020, "Di22"=4021, "Di23"=4022, "Di24"=4023, "Di_End"=4024, "ICU_End"=4025, "LedIllum"=10000, "ImicAxisXRel"=11000, "ImicAxisYRel"=11001, "ImicAxisZRel"=11002, "ImicAxisTurretRel"=11003, "ImicAxisFilter1Rel"=11004, "ImicAxisFilter2Rel"=11005, "ImicAxis_End"=11006, "ImicAxisXAbs"=11200, "ImicAxisYAbs"=11201, "ImicAxisZAbs"=11202, "ImicAxisTurretAbs"=11203, "ImicAxisFilter1Abs"=11204, "ImicAxisFilter2Abs"=11205, "ImicAxisXVel"=11300, "ImicAxisYVel"=11301, "ImicAxisZVel"=11302, "ImicAxisTurretVel"=11303, "ImicAxisFilter1Vel"=11304, "ImicAxisFilter2Vel"=11305, "ImicAxisXMoving"=11400, "ImicAxisYMoving"=11401, "ImicAxisZMoving"=11402, "ImicAxisTurretMoving"=11403, "ImicAxisFilter1Moving"=11404, "ImicAxisFilter2Moving"=11405, "ImicPiezoClip"=12001, "ImicPiezo"=12002, "IMIC_End"=12003] ("DeviceID")
                  # "LED:DA4:Range:0..5V\noder DO26=1025"
                  n63 = In Range and Coerce(upper limit=5.0 ("oberer Grenzwert"), x=w219, lower limit=-0.1 ("unterer Grenzwert")) -> (coerced(x)=w216:dbl)  [unwired: 1 out]
                  n64 = Bundle(cluster=w221, "Ring"=w220, "Value"=w216) -> (w222:cluster{"Ring":T2, "Value":dbl})
                }
                frame "led2" {
                  w223 = T2 1026 items=["EndLoop"=-2, "Loop"=-1, "Invalid"=0, "TriggerPolyV"=1, "TriggerCamera"=2, "SyncCamera"=3, "Do1"=1000, "Do2"=1001, "Do3"=1002, "Do4"=1003, "Do5"=1004, "Do6"=1005, "Do7"=1006, "Do8"=1007, "Do9"=1008, "Do10"=1009, "Do11"=1010, "Do12"=1011, "Do13"=1012, "Do14"=1013, "Do15"=1014, "Do16"=1015, "Do17"=1016, "Do18"=1017, "Do19"=1018, "Do20"=1019, "Do21"=1020, "Do22"=1021, "Do23"=1022, "Do24"=1023, "Do25"=1024, "Do26"=1025, "Do27"=1026, "Do28"=1027, "Do_End"=1028, "Da1"=2000, "Da2"=2001, "Da3"=2002, "Da4"=2003, "Da5"=2004, "Da6"=2005, "Da7"=2006, "Da8"=2007, "Da9"=2008, "Da10"=2009, "Da11"=2010, "Da12"=2011, "Da13"=2012, "Da14"=2013, "Da15"=2014, "Da16"=2015, "Da17"=2016, "Da18"=2017, "Da19"=2018, "DaLast"=2019, "Da1Incr"=2100, "Da2Incr"=2101, "Da3Incr"=2102, "Da4Incr"=2103, "Da5Incr"=2104, "Da6Incr"=2105, "Da7Incr"=2106, "Da8Incr"=2107, "Da1Raw"=2200, "Da2Raw"=2201, "Da3Raw"=2202, "Da4Raw"=2203, "Da5Raw"=2204, "Da6Raw"=2205, "Da7Raw"=2206, "Da8Raw"=2207, "Da1RawIncr"=2300, "Da2RawIncr"=2301, "Da3RawIncr"=2302, "Da4RawIncr"=2303, "Da5RawIncr"=2304, "Da6RawIncr"=2305, "Da7RawIncr"=2306, "Da8RawIncr"=2307, "Uart1"=3000, "Uart2"=3001, "Uart3"=3002, "Uart_End"=3003, "Di1"=4000, "Di2"=4001, "Di3"=4002, "Di4"=4003, "Di5"=4004, "Di6"=4005, "Di7"=4006, "Di8"=4007, "Di9"=4008, "Di10"=4009, "Di11"=4010, "Di12"=4011, "Di13"=4012, "Di14"=4013, "Di15"=4014, "Di16"=4015, "Di17"=4016, "Di18"=4017, "Di19"=4018, "Di20"=4019, "Di21"=4020, "Di22"=4021, "Di23"=4022, "Di24"=4023, "Di_End"=4024, "ICU_End"=4025, "LedIllum"=10000, "ImicAxisXRel"=11000, "ImicAxisYRel"=11001, "ImicAxisZRel"=11002, "ImicAxisTurretRel"=11003, "ImicAxisFilter1Rel"=11004, "ImicAxisFilter2Rel"=11005, "ImicAxis_End"=11006, "ImicAxisXAbs"=11200, "ImicAxisYAbs"=11201, "ImicAxisZAbs"=11202, "ImicAxisTurretAbs"=11203, "ImicAxisFilter1Abs"=11204, "ImicAxisFilter2Abs"=11205, "ImicAxisXVel"=11300, "ImicAxisYVel"=11301, "ImicAxisZVel"=11302, "ImicAxisTurretVel"=11303, "ImicAxisFilter1Vel"=11304, "ImicAxisFilter2Vel"=11305, "ImicAxisXMoving"=11400, "ImicAxisYMoving"=11401, "ImicAxisZMoving"=11402, "ImicAxisTurretMoving"=11403, "ImicAxisFilter1Moving"=11404, "ImicAxisFilter2Moving"=11405, "ImicPiezoClip"=12001, "ImicPiezo"=12002, "IMIC_End"=12003] ("Ring")
                  # "LED2 Range:0..5V\noder DO27=1026"
                  n65 = In Range and Coerce(upper limit=5.0 ("oberer Grenzwert"), x=w228, lower limit=-0.1 ("unterer Grenzwert")) -> (coerced(x)=w225:dbl)  [unwired: 1 out]
                  n66 = Bundle(cluster=w229, "Ring"=w223, "Value"=w225) -> (w230:cluster{"Ring":T2, "Value":dbl})
                }
                frame "led3" {
                  w231 = T2 1027 items=["EndLoop"=-2, "Loop"=-1, "Invalid"=0, "TriggerPolyV"=1, "TriggerCamera"=2, "SyncCamera"=3, "Do1"=1000, "Do2"=1001, "Do3"=1002, "Do4"=1003, "Do5"=1004, "Do6"=1005, "Do7"=1006, "Do8"=1007, "Do9"=1008, "Do10"=1009, "Do11"=1010, "Do12"=1011, "Do13"=1012, "Do14"=1013, "Do15"=1014, "Do16"=1015, "Do17"=1016, "Do18"=1017, "Do19"=1018, "Do20"=1019, "Do21"=1020, "Do22"=1021, "Do23"=1022, "Do24"=1023, "Do25"=1024, "Do26"=1025, "Do27"=1026, "Do28"=1027, "Do_End"=1028, "Da1"=2000, "Da2"=2001, "Da3"=2002, "Da4"=2003, "Da5"=2004, "Da6"=2005, "Da7"=2006, "Da8"=2007, "Da9"=2008, "Da10"=2009, "Da11"=2010, "Da12"=2011, "Da13"=2012, "Da14"=2013, "Da15"=2014, "Da16"=2015, "Da17"=2016, "Da18"=2017, "Da19"=2018, "DaLast"=2019, "Da1Incr"=2100, "Da2Incr"=2101, "Da3Incr"=2102, "Da4Incr"=2103, "Da5Incr"=2104, "Da6Incr"=2105, "Da7Incr"=2106, "Da8Incr"=2107, "Da1Raw"=2200, "Da2Raw"=2201, "Da3Raw"=2202, "Da4Raw"=2203, "Da5Raw"=2204, "Da6Raw"=2205, "Da7Raw"=2206, "Da8Raw"=2207, "Da1RawIncr"=2300, "Da2RawIncr"=2301, "Da3RawIncr"=2302, "Da4RawIncr"=2303, "Da5RawIncr"=2304, "Da6RawIncr"=2305, "Da7RawIncr"=2306, "Da8RawIncr"=2307, "Uart1"=3000, "Uart2"=3001, "Uart3"=3002, "Uart_End"=3003, "Di1"=4000, "Di2"=4001, "Di3"=4002, "Di4"=4003, "Di5"=4004, "Di6"=4005, "Di7"=4006, "Di8"=4007, "Di9"=4008, "Di10"=4009, "Di11"=4010, "Di12"=4011, "Di13"=4012, "Di14"=4013, "Di15"=4014, "Di16"=4015, "Di17"=4016, "Di18"=4017, "Di19"=4018, "Di20"=4019, "Di21"=4020, "Di22"=4021, "Di23"=4022, "Di24"=4023, "Di_End"=4024, "ICU_End"=4025, "LedIllum"=10000, "ImicAxisXRel"=11000, "ImicAxisYRel"=11001, "ImicAxisZRel"=11002, "ImicAxisTurretRel"=11003, "ImicAxisFilter1Rel"=11004, "ImicAxisFilter2Rel"=11005, "ImicAxis_End"=11006, "ImicAxisXAbs"=11200, "ImicAxisYAbs"=11201, "ImicAxisZAbs"=11202, "ImicAxisTurretAbs"=11203, "ImicAxisFilter1Abs"=11204, "ImicAxisFilter2Abs"=11205, "ImicAxisXVel"=11300, "ImicAxisYVel"=11301, "ImicAxisZVel"=11302, "ImicAxisTurretVel"=11303, "ImicAxisFilter1Vel"=11304, "ImicAxisFilter2Vel"=11305, "ImicAxisXMoving"=11400, "ImicAxisYMoving"=11401, "ImicAxisZMoving"=11402, "ImicAxisTurretMoving"=11403, "ImicAxisFilter1Moving"=11404, "ImicAxisFilter2Moving"=11405, "ImicPiezoClip"=12001, "ImicPiezo"=12002, "IMIC_End"=12003] ("Ring")
                  # "LED3:Range:0..5V\noder DO28=1027"
                  n67 = In Range and Coerce(upper limit=5.0 ("oberer Grenzwert"), x=w236, lower limit=-0.1 ("unterer Grenzwert")) -> (coerced(x)=w233:dbl)  [unwired: 1 out]
                  n68 = Bundle(cluster=w237, "Ring"=w231, "Value"=w233) -> (w238:cluster{"Ring":T2, "Value":dbl})
                }
                frame "led.intensity" {
                  w246 = 2016 items=["EndLoop"=-2, "Loop"=-1, "Invalid"=0, "TriggerPolyV"=1, "TriggerCamera"=2, "SyncCamera"=3, "Do1"=1000, "Do2"=1001, "Do3"=1002, "Do4"=1003, "Do5"=1004, "Do6"=1005, "Do7"=1006, "Do8"=1007, "Do9"=1008, "Do10"=1009, "Do11"=1010, "Do12"=1011, "Do13"=1012, "Do14"=1013, "Do15"=1014, "Do16"=1015, "Do17"=1016, "Do18"=1017, "Do19"=1018, "Do20"=1019, "Do21"=1020, "Do22"=1021, "Do23"=1022, "Do24"=1023, "Do_End"=1024, "Da1"=2000, "Da2"=2001, "Da3"=2002, "Da4"=2003, "Da5"=2004, "Da6"=2005, "Da7"=2006, "Da8"=2007, "Da17"=2016, "DaIncr_First"=2008, "Da1Incr"=2100, "Da2Incr"=2101, "Da3Incr"=2102, "Da4Incr"=2103, "Da5Incr"=2104, "Da6Incr"=2105, "Da7Incr"=2106, "Da8Incr"=2107, "Da1Raw"=2200, "Da2Raw"=2201, "Da3Raw"=2202, "Da4Raw"=2203, "Da5Raw"=2204, "Da6Raw"=2205, "Da7Raw"=2206, "Da8Raw"=2207, "Da1RawIncr"=2300, "Da2RawIncr"=2301, "Da3RawIncr"=2302, "Da4RawIncr"=2303, "Da5RawIncr"=2304, "Da6RawIncr"=2305, "Da7RawIncr"=2306, "Da8RawIncr"=2307, "Uart1"=3000, "Uart2"=3001, "Uart3"=3002, "Uart_End"=3003, "Di1"=4000, "Di2"=4001, "Di3"=4002, "Di4"=4003, "Di5"=4004, "Di6"=4005, "Di7"=4006, "Di8"=4007, "Di9"=4008, "Di10"=4009, "Di11"=4010, "Di12"=4011, "Di13"=4012, "Di14"=4013, "Di15"=4014, "Di16"=4015, "Di17"=4016, "Di18"=4017, "Di19"=4018, "Di20"=4019, "Di21"=4020, "Di22"=4021, "Di23"=4022, "Di24"=4023, "Di_End"=4024, "ICU_End"=4025, "LedIllum"=10000, "ImicAxisXRel"=11000, "ImicAxisYRel"=11001, "ImicAxisZRel"=11002, "ImicAxisTurretRel"=11003, "ImicAxisFilter1Rel"=11004, "ImicAxisFilter2Rel"=11005, "ImicAxis_End"=11006, "ImicAxisXAbs"=11200, "ImicAxisYAbs"=11201, "ImicAxisZAbs"=11202, "ImicAxisTurretAbs"=11203, "ImicAxisFilter1Abs"=11204, "ImicAxisFilter2Abs"=11205, "ImicAxisXVel"=11300, "ImicAxisYVel"=11301, "ImicAxisZVel"=11302, "ImicAxisTurretVel"=11303, "ImicAxisFilter1Vel"=11304, "ImicAxisFilter2Vel"=11305, "ImicAxisXMoving"=11400, "ImicAxisYMoving"=11401, "ImicAxisZMoving"=11402, "ImicAxisTurretMoving"=11403, "ImicAxisFilter1Moving"=11404, "ImicAxisFilter2Moving"=11405, "ImicPiezoClip"=12001, "ImicPiezo"=12002, "IMIC_End"=12003] ("DeviceID")
                  n69 = In Range and Coerce(upper limit=5.0 ("oberer Grenzwert"), x=w243, lower limit=0.0 ("unterer Grenzwert")) -> (coerced(x)=w242:dbl)  [unwired: 1 out]
                  n70 = Bundle(cluster=w240, "Ring"=w246, "Value"=w242) -> (w241:cluster{"Ring":T2, "Value":dbl})
                }
                frame "led2.intensity" {
                  w254 = 2017 items=["EndLoop"=-2, "Loop"=-1, "Invalid"=0, "TriggerPolyV"=1, "TriggerCamera"=2, "SyncCamera"=3, "Do1"=1000, "Do2"=1001, "Do3"=1002, "Do4"=1003, "Do5"=1004, "Do6"=1005, "Do7"=1006, "Do8"=1007, "Do9"=1008, "Do10"=1009, "Do11"=1010, "Do12"=1011, "Do13"=1012, "Do14"=1013, "Do15"=1014, "Do16"=1015, "Do17"=1016, "Do18"=1017, "Do19"=1018, "Do20"=1019, "Do21"=1020, "Do22"=1021, "Do23"=1022, "Do24"=1023, "Do_End"=1024, "Da1"=2000, "Da2"=2001, "Da3"=2002, "Da4"=2003, "Da5"=2004, "Da6"=2005, "Da7"=2006, "Da8"=2007, "Da17"=2016, "Da18"=2017, "Da19"=2018, "DaIncr_First"=2008, "Da1Incr"=2100, "Da2Incr"=2101, "Da3Incr"=2102, "Da4Incr"=2103, "Da5Incr"=2104, "Da6Incr"=2105, "Da7Incr"=2106, "Da8Incr"=2107, "Da1Raw"=2200, "Da2Raw"=2201, "Da3Raw"=2202, "Da4Raw"=2203, "Da5Raw"=2204, "Da6Raw"=2205, "Da7Raw"=2206, "Da8Raw"=2207, "Da1RawIncr"=2300, "Da2RawIncr"=2301, "Da3RawIncr"=2302, "Da4RawIncr"=2303, "Da5RawIncr"=2304, "Da6RawIncr"=2305, "Da7RawIncr"=2306, "Da8RawIncr"=2307, "Uart1"=3000, "Uart2"=3001, "Uart3"=3002, "Uart_End"=3003, "Di1"=4000, "Di2"=4001, "Di3"=4002, "Di4"=4003, "Di5"=4004, "Di6"=4005, "Di7"=4006, "Di8"=4007, "Di9"=4008, "Di10"=4009, "Di11"=4010, "Di12"=4011, "Di13"=4012, "Di14"=4013, "Di15"=4014, "Di16"=4015, "Di17"=4016, "Di18"=4017, "Di19"=4018, "Di20"=4019, "Di21"=4020, "Di22"=4021, "Di23"=4022, "Di24"=4023, "Di_End"=4024, "ICU_End"=4025, "LedIllum"=10000, "ImicAxisXRel"=11000, "ImicAxisYRel"=11001, "ImicAxisZRel"=11002, "ImicAxisTurretRel"=11003, "ImicAxisFilter1Rel"=11004, "ImicAxisFilter2Rel"=11005, "ImicAxis_End"=11006, "ImicAxisXAbs"=11200, "ImicAxisYAbs"=11201, "ImicAxisZAbs"=11202, "ImicAxisTurretAbs"=11203, "ImicAxisFilter1Abs"=11204, "ImicAxisFilter2Abs"=11205, "ImicAxisXVel"=11300, "ImicAxisYVel"=11301, "ImicAxisZVel"=11302, "ImicAxisTurretVel"=11303, "ImicAxisFilter1Vel"=11304, "ImicAxisFilter2Vel"=11305, "ImicAxisXMoving"=11400, "ImicAxisYMoving"=11401, "ImicAxisZMoving"=11402, "ImicAxisTurretMoving"=11403, "ImicAxisFilter1Moving"=11404, "ImicAxisFilter2Moving"=11405, "ImicPiezoClip"=12001, "ImicPiezo"=12002, "IMIC_End"=12003] ("DeviceID")
                  n71 = In Range and Coerce(upper limit=5.0 ("oberer Grenzwert"), x=w251, lower limit=0.0 ("unterer Grenzwert")) -> (coerced(x)=w250:dbl)  [unwired: 1 out]
                  n72 = Bundle(cluster=w248, "Ring"=w254, "Value"=w250) -> (w249:cluster{"Ring":T2, "Value":dbl})
                }
                frame "led3.intensity" {
                  w255 = T2 2018 items=["EndLoop"=-2, "Loop"=-1, "Invalid"=0, "TriggerPolyV"=1, "TriggerCamera"=2, "SyncCamera"=3, "Do1"=1000, "Do2"=1001, "Do3"=1002, "Do4"=1003, "Do5"=1004, "Do6"=1005, "Do7"=1006, "Do8"=1007, "Do9"=1008, "Do10"=1009, "Do11"=1010, "Do12"=1011, "Do13"=1012, "Do14"=1013, "Do15"=1014, "Do16"=1015, "Do17"=1016, "Do18"=1017, "Do19"=1018, "Do20"=1019, "Do21"=1020, "Do22"=1021, "Do23"=1022, "Do24"=1023, "Do25"=1024, "Do26"=1025, "Do27"=1026, "Do28"=1027, "Do_End"=1028, "Da1"=2000, "Da2"=2001, "Da3"=2002, "Da4"=2003, "Da5"=2004, "Da6"=2005, "Da7"=2006, "Da8"=2007, "Da9"=2008, "Da10"=2009, "Da11"=2010, "Da12"=2011, "Da13"=2012, "Da14"=2013, "Da15"=2014, "Da16"=2015, "Da17"=2016, "Da18"=2017, "Da19"=2018, "DaLast"=2019, "Da1Incr"=2100, "Da2Incr"=2101, "Da3Incr"=2102, "Da4Incr"=2103, "Da5Incr"=2104, "Da6Incr"=2105, "Da7Incr"=2106, "Da8Incr"=2107, "Da1Raw"=2200, "Da2Raw"=2201, "Da3Raw"=2202, "Da4Raw"=2203, "Da5Raw"=2204, "Da6Raw"=2205, "Da7Raw"=2206, "Da8Raw"=2207, "Da1RawIncr"=2300, "Da2RawIncr"=2301, "Da3RawIncr"=2302, "Da4RawIncr"=2303, "Da5RawIncr"=2304, "Da6RawIncr"=2305, "Da7RawIncr"=2306, "Da8RawIncr"=2307, "Uart1"=3000, "Uart2"=3001, "Uart3"=3002, "Uart_End"=3003, "Di1"=4000, "Di2"=4001, "Di3"=4002, "Di4"=4003, "Di5"=4004, "Di6"=4005, "Di7"=4006, "Di8"=4007, "Di9"=4008, "Di10"=4009, "Di11"=4010, "Di12"=4011, "Di13"=4012, "Di14"=4013, "Di15"=4014, "Di16"=4015, "Di17"=4016, "Di18"=4017, "Di19"=4018, "Di20"=4019, "Di21"=4020, "Di22"=4021, "Di23"=4022, "Di24"=4023, "Di_End"=4024, "ICU_End"=4025, "LedIllum"=10000, "ImicAxisXRel"=11000, "ImicAxisYRel"=11001, "ImicAxisZRel"=11002, "ImicAxisTurretRel"=11003, "ImicAxisFilter1Rel"=11004, "ImicAxisFilter2Rel"=11005, "ImicAxis_End"=11006, "ImicAxisXAbs"=11200, "ImicAxisYAbs"=11201, "ImicAxisZAbs"=11202, "ImicAxisTurretAbs"=11203, "ImicAxisFilter1Abs"=11204, "ImicAxisFilter2Abs"=11205, "ImicAxisXVel"=11300, "ImicAxisYVel"=11301, "ImicAxisZVel"=11302, "ImicAxisTurretVel"=11303, "ImicAxisFilter1Vel"=11304, "ImicAxisFilter2Vel"=11305, "ImicAxisXMoving"=11400, "ImicAxisYMoving"=11401, "ImicAxisZMoving"=11402, "ImicAxisTurretMoving"=11403, "ImicAxisFilter1Moving"=11404, "ImicAxisFilter2Moving"=11405, "ImicPiezoClip"=12001, "ImicPiezo"=12002, "IMIC_End"=12003] ("Ring")
                  n73 = In Range and Coerce(upper limit=5.0 ("oberer Grenzwert"), x=w260, lower limit=0.0 ("unterer Grenzwert")) -> (coerced(x)=w259:dbl)  [unwired: 1 out]
                  n74 = Bundle(cluster=w257, "Ring"=w255, "Value"=w259) -> (w258:cluster{"Ring":T2, "Value":dbl})
                }
              }
              n75 = case shown="No Error" w109 {
                selector: w109 -> [w269 w282]
                tunnel: [w268 w282] -> w113
                tunnel: w107 -> [w271 _]
                tunnel: w110 -> [w265 _]
                tunnel: w108 -> [w267 _]
                tunnel: w105 -> [w266 _]
                frame No Error {
                  n76 = Unbundle(w265) -> ("Ring"=w264:T2, "Value"=w263:dbl)
                  n77 = call "IMIC_SetDevice.vi"("Value"=w263, "DeviceID"=w264, "handle"=w271) -> ("output param"=w270:T3)  [unwired: 1 out]
                  n78 = case shown="\"no error\"" w270 {
                    selector: w270 -> [_ w279]
                    tunnel: w269 -> [w277 _]
                    tunnel: [w277 w281] -> w268
                    tunnel: w267 -> [w273 _]
                    tunnel: w266 -> [w272 _]
                    frame "no error" {
                      n79 = Number To Engineering String(1:FALSE ("use system decimal point (T)"), 4:w272) -> (0:w276:string)  [unwired: 2 out]
                      n80 = call "Variables.vi"("value"=w276, "Tag in"=w273, "Command"=T1."ChangeValue") -> ()  [unwired: 3 out]
                    }
                    frame "missing axis", Default {
                      # "sdk error"
                      n81 = Format Into String(w279) -> (resulting string=w278:string)  [unwired: 3 in, 1 out]
                      n82 = Bundle(TRUE, "output param"=w279, w278) -> (w281:T4)  [unwired: 1 out]
                    }
                  }
                }
                frame Error {
                }
              }
            }
          }
          "error out" <- w32
          n83 = call "ErrorLog.vi"("error in (no error)"=w32) -> ()  [unwired: 2 out]
        }
        n84 = Unbundle By Name(w27) -> ("status"=w31:bool)
      }
      n85 = call "IMIC_IsInit.vi"("handle"=w10) -> ("output param"=w11:T3, "handle out"=w9:u64)  [unwired: 1 out]
      n86 = case shown="\"no error\"" w11 {
        selector: w11 -> [_ w23]
        tunnel: [w22 w23] -> _
        tunnel: w9 -> [w21 _]
        frame "no error" {
          n87 = call "IMIC_Close.vi"("handle"=w21) -> ("output param"=w22:T3)  [unwired: 1 out]
        }
        frame "wrong handle", Default {
        }
      }
    }
    frame Error {
    }
  }
